vi "Zero_padding.vi"() -> ()   [LabVIEW 2009]
uses:
  <vilib>/imath/engines/lvmath2/RunTimeEngine/ErrorHandling/NIMS_Finalize Error.vi
  <vilib>/imath/engines/lvmath2/RunTimeEngine/Parser/MC_Version.vi
  <vilib>/imath/engines/lvmath2/RunTimeEngine/NodeEndStatement/NIMS_NodeEndStatement_Output.vi
  <instcachedir>/0/NIMS_NodeEndStatement_Output_53EC0D466D134D7ABD903AC30B43404B.lvgen/NIMS_NodeEndStatement_Output_53EC0D466D134D7ABD903AC30B43404B_001.vi
  <vilib>/imath/engines/lvmath/Functions/Error Handling/MergeErrorsWrapper.vi
  <vilib>/imath/engines/lvmath2/RunTimeEngine/NodeEndStatement/NIMS_NodeEndStatement_Get Vector.vi
  <instcachedir>/0/NIMS_NodeEndStatement_Get Vector_708AE642CFEE4B9892E482CBBBA3A4D6.lvgen/NIMS_NodeEndStatement_Get Vector_708AE642CFEE4B9892E482CBBBA3A4D6_000.vi
  <vilib>/imath/engines/lvmath2/RunTimeEngine/RangeToken/NIMS_Range.vi
  <instcachedir>/0/NIMS_Range_08574DECC23E450FAF0AC0BC39E6BEA7.lvgen/NIMS_Range_08574DECC23E450FAF0AC0BC39E6BEA7_000.vi
  <vilib>/imathl/engines/lvmath/Functions/Error Handling/Create Error.vi
  <vilib>/imath/engines/lvmath/Functions/Error Handling/MC_Error Cluster From Error Code.vi
  <vilib>/imath/engines/lvmath2/RunTimeEngine/BuiltInFunctions/abs/NIMS_abs(signed).vi
  <instcachedir>/0/NIMS_abs(signed)_C4FCB8E6058B49B797C7C8D53CA5F6EC.lvgen/NIMS_abs(signed)_C4FCB8E6058B49B797C7C8D53CA5F6EC_000.vi
  <vilib>/imath/engines/lvmath2/RunTimeEngine/BuiltInFunctions/fft/NIMS_fft(GV).vi
  <instcachedir>/0/NIMS_fft(GV)_4C6467FC22F84E4BA42517A07EF978B0.lvgen/NIMS_fft(GV)_4C6467FC22F84E4BA42517A07EF978B0_001.vi
  <vilib>/imath/engines/lvmath2/RunTimeEngine/BuiltInFunctions/zeros/NIMS_M=zeros(I32).vi
  <vilib>/imath/engines/lvmath2/RunTimeEngine/ReplaceToken/NIMS_Replace - Assignment Check _(_)=VorM.vi
  <instcachedir>/0/NIMS_Replace - Assignment Check _(_)=VorM_38617C4B4BE24F7B8590CF2FBC0C8111.lvgen/NIMS_Replace - Assignment Check _(_)=VorM_38617C4B4BE24F7B8590CF2FBC0C8111_005.vi
  <vilib>/imath/engines/lvmath2/RunTimeEngine/ReplaceToken/NIMS_Replace - Size Check _(_)=VorM.vi
  <instcachedir>/0/NIMS_Replace - Size Check _(_)=VorM_06A8B9059C234BF590D22CF9E7D69236.lvgen/NIMS_Replace - Size Check _(_)=VorM_06A8B9059C234BF590D22CF9E7D69236_005.vi
  <vilib>/imath/engines/lvmath2/RunTimeEngine/VariableToken/Read/NIMS_Get Elements - RV(_) - Check.vi
  <instcachedir>/0/NIMS_Get Elements - RV(_) - Check_30A5434E2C4242B098C990FE3FB371BC.lvgen/NIMS_Get Elements - RV(_) - Check_30A5434E2C4242B098C990FE3FB371BC_003.vi
  <vilib>/imath/engines/lvmath2/RunTimeEngine/RangeToken/NIMS_Range_R2.vi
  <vilib>/imath/engines/lvmath2/RunTimeEngine/ReplaceToken/NIMS_Replace - Check Linear.vi
  <instcachedir>/0/NIMS_Replace - Check Linear_3F5099154F904E698C6642037B8E50AB.lvgen/NIMS_Replace - Check Linear_3F5099154F904E698C6642037B8E50AB_005.vi
  <instcachedir>/0/NIMS_abs(signed)_C4FCB8E6058B49B797C7C8D53CA5F6EC.lvgen/NIMS_abs(signed)_C4FCB8E6058B49B797C7C8D53CA5F6EC_002.vi
  <vilib>/imath/engines/lvmath2/RunTimeEngine/BuiltInFunctions/fft/NIMS_fft(GM).vi
  <instcachedir>/0/NIMS_fft(GM)_D61006EB97DF48D4B7BC0A22887DF931.lvgen/NIMS_fft(GM)_D61006EB97DF48D4B7BC0A22887DF931_000.vi
panel:
  out "Frequency 128":dbl[](graph)
  out "Time 128":dbl[](graph)
  out "Frequency 64":dbl[](graph)
  out "Time 64":dbl[](graph)
  out "Frequency 32":dbl[](graph)
  out "Time 32":dbl[](graph)
  out "Frequency 16":dbl[](graph)
  out "Time 16":dbl[](graph)
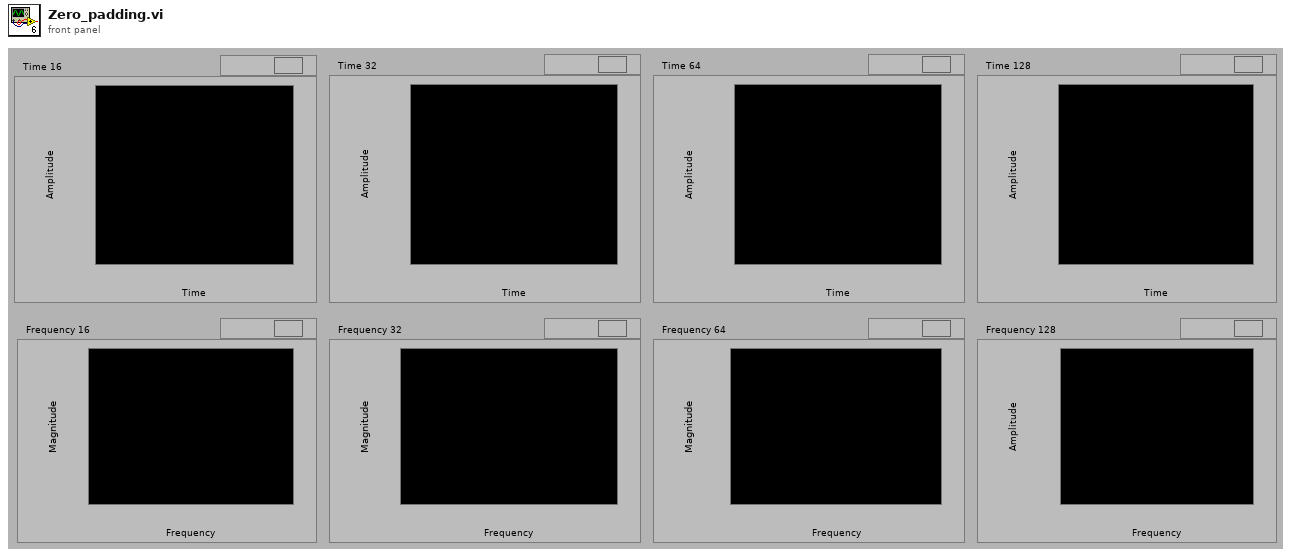
[diagram p1: front panel]
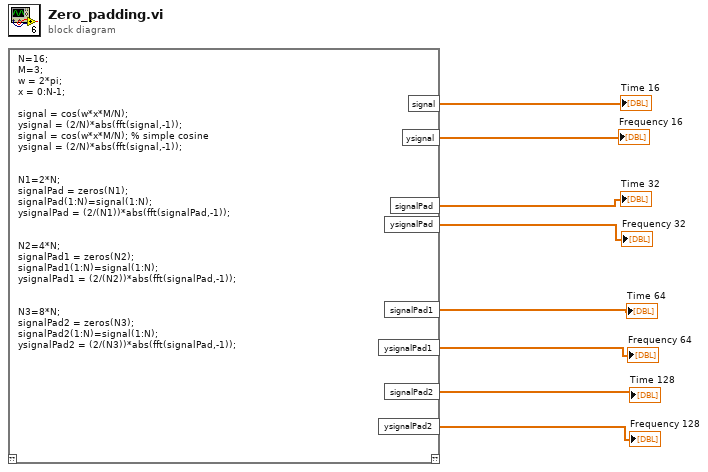
[diagram p0: block diagram]
diagram:
  n1 = mathscript code="N=16;\nM=3;\nw = 2*pi;\nx = 0:N-1;\n\nsignal = cos(w*x*M/N);\nysignal = (2/N)*abs(fft(signal,-1));\nsignal = cos(w*x*M/N); % simple cosine\nysignal = (2/N)*abs(fft(signal,-1));\n\n\nN1=2*N;\nsignalPad = zeros(N1);\nsignalPad(1:N)=signal(1:N);\nysignalPad = (2/(N1))*abs(fft(signalPad,-1));\n\n\nN2=4*N;\nsignalPad1 = zeros(N2);\nsignalPad1(1:N)=signal(1:N);\nysignalPad1 = (2/(N2))*abs(fft(signalPad,-1));\n\n\nN3=8*N;\nsignalPad2 = zeros(N3);\nsignalPad2(1:N)=signal(1:N);\nysignalPad2 = (2/(N3))*abs(fft(signalPad,-1));"() -> ("signal"=→"Time 16":dbl[], "ysignal"=→"Frequency 16":dbl[], "signalPad"=→"Time 32":dbl[], "ysignalPad"=→"Frequency 32":dbl[], "signalPad1"=→"Time 64":dbl[], "ysignalPad1"=→"Frequency 64":dbl[], "signalPad2"=→"Time 128":dbl[], "ysignalPad2"=→"Frequency 128":dbl[])  [unwired: 1 in, 1 out]
